vi "Main_old.vi"() -> ()   [LabVIEW 2021]
uses:
  Enums/States_Enum.ctl
panel:
  in  "voltage":dbl
  out "Battery Inserted":bool
  in  "stop":bool
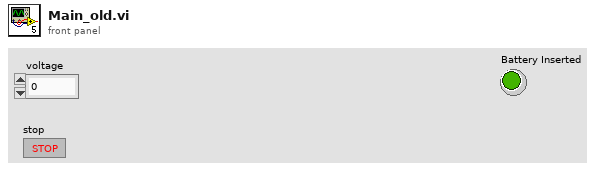
[diagram p1: front panel]
types:
  T1 = typedef "States_Enum.ctl" = enum16{"No_Battery", "Battery_Inserted", ""}
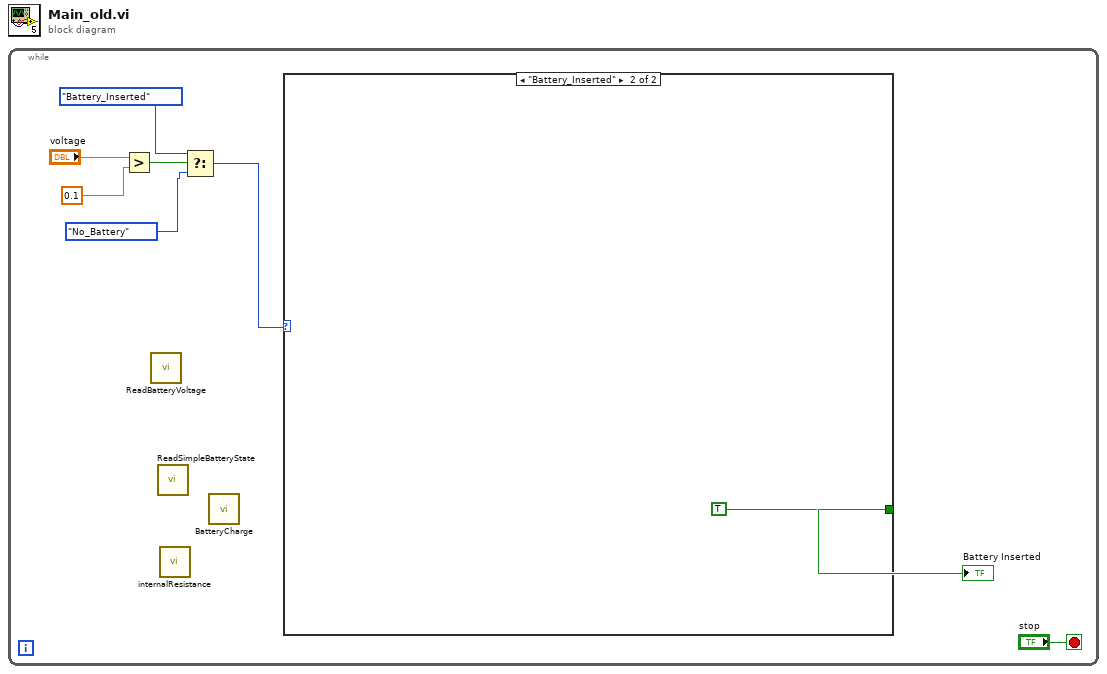
[diagram p0: block diagram]
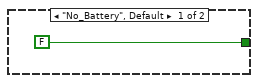
[diagram p2: hidden frame]
diagram:
  n1 = while {
    stop <- "stop" stop-if-true
    n2 = Greater?(x="voltage", y=0.1) -> (0:w7:bool)
    n3 = call "ReadBatteryVoltage.vi"() -> ()  [unwired: 8 in, 4 out]
    n4 = call "ReadSimpleBatteryState.vi"() -> ()  [unwired: 10 in, 2 out]
    n5 = call "internalResistance.vi"() -> ()  [unwired: 11 in, 1 out]
    n6 = Select(t=States_Enum."Battery_Inserted", s=w7, f=States_Enum."No_Battery") -> (s? t:f=w3:T1)
    n7 = call "BatteryCharge.vi"() -> ()  [unwired: 11 in, 1 out]
    n8 = case shown="\"Battery_Inserted\"" w3 {
      tunnel: [FALSE TRUE] -> w1
      frame "No_Battery", Default {
      }
      frame "Battery_Inserted" {
      }
    }
    "Battery Inserted" <- w1
  }
